vi "Interval timer.vi"(9 "Interval [s]":dbl) -> (1 "Timer value [s]":dbl)   [LabVIEW 2017]
panel:
  out "Error Out":errorcluster
  in  "Error In":errorcluster
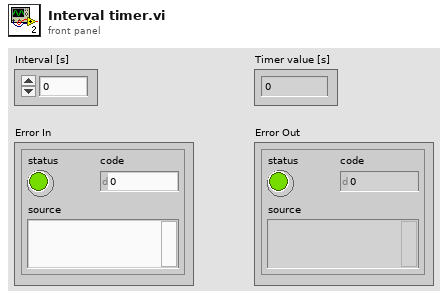
[diagram p1: front panel]
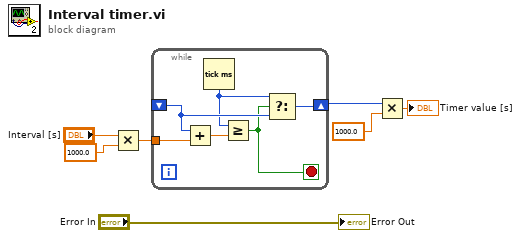
[diagram p0: block diagram]
diagram:
  n1 = Multiply(x="Interval [s]", y=1000.0) -> (x*y=w1:dbl)
  n2 = while {
    shift-right: [w9] -> w6
    shift-left: _ -> [w12]
    tunnel: w1 -> [w8]
    stop <- w11 stop-if-true
    n3 = Add(x=w12, y=w8) -> (x+y=w13:dbl)
    n4 = Tick Count (ms)() -> (millisecond timer value=w10:u32)
    n5 = Greater Or Equal?(x=w10, y=w13) -> (x >= y?=w11:bool)
    n6 = Select(t=w10, s=w11, f=w12) -> (s? t:f=w9:u32)
  }
  n7 = Multiply(x=w6, y=1000.0) -> (x*y=→"Timer value [s]":dbl)
  "Error Out" <- "Error In"
